vi "Feature Step Call.vi"(11 "Feature List (In)":T2(array[cluster])=[{"Item Name"="test1", "Item Status"=TRUE, "Steps"=[{"Channel Type"="C", "Channels"="6:", "Wait/Poll (ms)"=100, "Parameter"=2, "STM-Speed"=0, "STM-Degree"=0, "Direction"=0}, {"Channel Type"="N", "Channels"="", "Wait/Poll (ms)"=100, "Parameter"=0, "STM-Speed"=0, "STM-Degree"=0, "Direction"=0}, {"Channel Type"="C", "Channels"="6:", "Wait/Poll (ms)"=100, "Parameter"=1, "STM-Speed"=0, "STM-Degree"=0, "Direction"=0}, {"Channel Type"="C", "Channels"="7:", "Wait/Poll (ms)"=100, "Parameter"=2, "STM-Speed"=0, "STM-Degree"=0, "Direction"=0}, {"Channel Type"="C", "Channels"="8:", "Wait/Poll (ms)"=100, "Parameter"=2, "STM-Speed"=0, "STM-Degree"=0, "Direction"=0}, {"Channel Type"="C", "Channels"="7:", "Wait/Poll (ms)"=100, "Parameter"=1, "STM-Speed"=0, "STM-Degree"=0, "Direction"=0}, {"Channel Type"="N", "Channels"="", "Wait/Poll (ms)"=100, "Parameter"=0, "STM-Speed"=0, "STM-Degree"=0, "Direction"=0}]}, {"Item Name"="test2", "Item Status"=TRUE, "Steps"=[{"Channel Type"="C", "Channels"="11:", "Wait/Poll (ms)"=100, "Parameter"=2, "STM-Speed"=0, "STM-Degree"=0, "Direction"=0}, {"Channel Type"="C", "Channels"="12:", "Wait/Poll (ms)"=100, "Parameter"=1, "STM-Speed"=0, "STM-Degree"=0, "Direction"=0}, {"Channel Type"="C", "Channels"="12:", "Wait/Poll (ms)"=100, "Parameter"=2, "STM-Speed"=0, "STM-Degree"=0, "Direction"=0}, {"Channel Type"="C", "Channels"="12:", "Wait/Poll (ms)"=100, "Parameter"=1, "STM-Speed"=0, "STM-Degree"=0, "Direction"=0}, {"Channel Type"="N", "Channels"="", "Wait/Poll (ms)"=100, "Parameter"=0, "STM-Speed"=0, "STM-Degree"=0, "Direction"=0}]}]) -> (0 "Feature Step":string[][](array[string]), 1 "Feature list out":T2(array[cluster]))   [LabVIEW 2015]
uses:
  Galobal variable_TI.vi
panel:
  out "Channels (Out)":i32[](array[numeric])
  out "Channels":string
  out "Feature list out 2":T1(array[cluster])=[{"Item Name"="Winker", "Item Status"=TRUE, "Steps"=[{"Channel Type"="C", "Channels"="3:", "Wait/Poll (ms)"=0, "Parameter"=2, "STM-Speed"=0, "STM-Degree"=0, "Direction"=0}, {"Channel Type"="N", "Channels"="", "Wait/Poll (ms)"=500, "Parameter"=0, "STM-Speed"=0, "STM-Degree"=0, "Direction"=0}, {"Channel Type"="AI", "Channels"="5:", "Wait/Poll (ms)"=1000, "Parameter"=2, "STM-Speed"=0, "STM-Degree"=0, "Direction"=0}, {"Channel Type"="AI", "Channels"="0:", "Wait/Poll (ms)"=1000, "Parameter"=2, "STM-Speed"=0, "STM-Degree"=0, "Direction"=0}, {"Channel Type"="N", "Channels"="", "Wait/Poll (ms)"=500, "Parameter"=0, "STM-Speed"=0, "STM-Degree"=0, "Direction"=0}, {"Channel Type"="C", "Channels"="3:", "Wait/Poll (ms)"=0, "Parameter"=1, "STM-Speed"=0, "STM-Degree"=0, "Direction"=0}, {"Channel Type"="N", "Channels"="", "Wait/Poll (ms)"=500, "Parameter"=0, "STM-Speed"=0, "STM-Degree"=0, "Direction"=0}, {"Channel Type"="N", "Channels"="", "Wait/Poll (ms)"=500, "Parameter"=0, "STM-Speed"=0, "STM-Degree"=0, "Direction"=0}, {"Channel Type"="C", "Channels"="5:", "Wait/Poll (ms)"=0, "Parameter"=2, "STM-Speed"=0, "STM-Degree"=0, "Direction"=0}, {"Channel Type"="C", "Channels"="5:", "Wait/Poll (ms)"=0, "Parameter"=1, "STM-Speed"=0, "STM-Degree"=0, "Direction"=0}, {"Channel Type"="N", "Channels"="", "Wait/Poll (ms)"=500, "Parameter"=0, "STM-Speed"=0, "STM-Degree"=0, "Direction"=0}, {"Channel Type"="N", "Channels"="", "Wait/Poll (ms)"=500, "Parameter"=0, "STM-Speed"=0, "STM-Degree"=0, "Direction"=0}, {"Channel Type"="N", "Channels"="", "Wait/Poll (ms)"=500, "Parameter"=0, "STM-Speed"=0, "STM-Degree"=0, "Direction"=0}, {"Channel Type"="C", "Channels"="4:", "Wait/Poll (ms)"=0, "Parameter"=2, "STM-Speed"=0, "STM-Degree"=0, "Direction"=0}, {"Channel Type"="N", "Channels"="", "Wait/Poll (ms)"=500, "Parameter"=0, "STM-Speed"=0, "STM-Degree"=0, "Direction"=0}, {"Channel Type"="AI", "Channels"="4:", "Wait/Poll (ms)"=1000, "Parameter"=2, "STM-Speed"=0, "STM-Degree"=0, "Direction"=0}, {"Channel Type"="AI", "Channels"="0:", "Wait/Poll (ms)"=1000, "Parameter"=2, "STM-Speed"=0, "STM-Degree"=0, "Direction"=0}, {"Channel Type"="N", "Channels"="", "Wait/Poll (ms)"=500, "Parameter"=0, "STM-Speed"=0, "STM-Degree"=0, "Direction"=0}, {"Channel Type"="C", "Channels"="4:", "Wait/Poll (ms)"=0, "Parameter"=1, "STM-Speed"=0, "STM-Degree"=0, "Direction"=0}, {"Channel Type"="N", "Channels"="", "Wait/Poll (ms)"=500, "Parameter"=0, "STM-Speed"=0, "STM-Degree"=0, "Direction"=0}, {"Channel Type"="N", "Channels"="", "Wait/Poll (ms)"=500, "Parameter"=0, "STM-Speed"=0, "STM-Degree"=0, "Direction"=0}, {"Channel Type"="C", "Channels"="5:", "Wait/Poll (ms)"=0, "Parameter"=2, "STM-Speed"=0, "STM-Degree"=0, "Direction"=0}, {"Channel Type"="N", "Channels"="", "Wait/Poll (ms)"=500, "Parameter"=0, "STM-Speed"=0, "STM-Degree"=0, "Direction"=0}, {"Channel Type"="N", "Channels"="", "Wait/Poll (ms)"=500, "Parameter"=0, "STM-Speed"=0, "STM-Degree"=0, "Direction"=0}, {"Channel Type"="C", "Channels"="5:", "Wait/Poll (ms)"=0, "Parameter"=1, "STM-Speed"=0, "STM-Degree"=0, "Direction"=0}, {"Channel Type"="N", "Channels"="", "Wait/Poll (ms)"=500, "Parameter"=0, "STM-Speed"=0, "STM-Degree"=0, "Direction"=0}, {"Channel Type"="N", "Channels"="", "Wait/Poll (ms)"=500, "Parameter"=0, "STM-Speed"=0, "STM-Degree"=0, "Direction"=0}]}, {"Item Name"="Horn", "Item Status"=TRUE, "Steps"=[{"Channel Type"="C", "Channels"="8:", "Wait/Poll (ms)"=0, "Parameter"=2, "STM-Speed"=0, "STM-Degree"=0, "Direction"=0}, {"Channel Type"="N", "Channels"="", "Wait/Poll (ms)"=500, "Parameter"=0, "STM-Speed"=0, "STM-Degree"=0, "Direction"=0}, {"Channel Type"="AI", "Channels"="9:", "Wait/Poll (ms)"=1000, "Parameter"=2, "STM-Speed"=0, "STM-Degree"=0, "Direction"=0}, {"Channel Type"="AI", "Channels"="3:", "Wait/Poll (ms)"=1000, "Parameter"=2, "STM-Speed"=0, "STM-Degree"=0, "Direction"=0}, {"Channel Type"="N", "Channels"="", "Wait/Poll (ms)"=500, "Parameter"=0, "STM-Speed"=0, "STM-Degree"=0, "Direction"=0}, {"Channel Type"="C", "Channels"="8:", "Wait/Poll (ms)"=0, "Parameter"=1, "STM-Speed"=0, "STM-Degree"=0, "Direction"=0}, {"Channel Type"="N", "Channels"="", "Wait/Poll (ms)"=500, "Parameter"=0, "STM-Speed"=0, "STM-Degree"=0, "Direction"=0}, {"Channel Type"="N", "Channels"="", "Wait/Poll (ms)"=500, "Parameter"=0, "STM-Speed"=0, "STM-Degree"=0, "Direction"=0}]}, {"Item Name"="Passing", "Item Status"=TRUE, "Steps"=[{"Channel Type"="C", "Channels"="8:", "Wait/Poll (ms)"=0, "Parameter"=2, "STM-Speed"=0, "STM-Degree"=0, "Direction"=0}, {"Channel Type"="N", "Channels"="", "Wait/Poll (ms)"=500, "Parameter"=0, "STM-Speed"=0, "STM-Degree"=0, "Direction"=0}, {"Channel Type"="C", "Channels"="8:", "Wait/Poll (ms)"=0, "Parameter"=1, "STM-Speed"=0, "STM-Degree"=0, "Direction"=0}, {"Channel Type"="N", "Channels"="", "Wait/Poll (ms)"=500, "Parameter"=0, "STM-Speed"=0, "STM-Degree"=0, "Direction"=0}]}, {"Item Name"="-1", "Item Status"=FALSE, "Steps"=[]}, {"Item Name"="-1", "Item Status"=FALSE, "Steps"=[]}, {"Item Name"="-1", "Item Status"=FALSE, "Steps"=[]}, {"Item Name"="-1", "Item Status"=FALSE, "Steps"=[]}, {"Item Name"="Screw ", "Item Status"=TRUE, "Steps"=[{"Channel Type"="C", "Channels"="1:", "Wait/Poll (ms)"=1000, "Parameter"=1, "STM-Speed"=0, "STM-Degree"=0, "Direction"=0}, {"Channel Type"="F", "Channels"="12:", "Wait/Poll (ms)"=1000, "Parameter"=1, "STM-Speed"=0, "STM-Degree"=0, "Direction"=0}, {"Channel Type"="C", "Channels"="0:", "Wait/Poll (ms)"=1000, "Parameter"=2, "STM-Speed"=0, "STM-Degree"=0, "Direction"=0}, {"Channel Type"="N", "Channels"="", "Wait/Poll (ms)"=200, "Parameter"=0, "STM-Speed"=0, "STM-Degree"=0, "Direction"=0}, {"Channel Type"="F", "Channels"="12:", "Wait/Poll (ms)"=1000, "Parameter"=2, "STM-Speed"=0, "STM-Degree"=0, "Direction"=0}, {"Channel Type"="N", "Channels"="", "Wait/Poll (ms)"=200, "Parameter"=0, "STM-Speed"=0, "STM-Degree"=0, "Direction"=0}, {"Channel Type"="C", "Channels"="0:", "Wait/Poll (ms)"=0, "Parameter"=1, "STM-Speed"=0, "STM-Degree"=0, "Direction"=0}, {"Channel Type"="N", "Channels"="", "Wait/Poll (ms)"=100, "Parameter"=0, "STM-Speed"=0, "STM-Degree"=0, "Direction"=0}]}, {"Item Name"="Stamping", "Item Status"=TRUE, "Steps"=[{"Channel Type"="C", "Channels"="5:", "Wait/Poll (ms)"=1000, "Parameter"=2, "STM-Speed"=0, "STM-Degree"=0, "Direction"=0}, {"Channel Type"="N", "Channels"="", "Wait/Poll (ms)"=200, "Parameter"=0, "STM-Speed"=0, "STM-Degree"=0, "Direction"=0}, {"Channel Type"="F", "Channels"="13:", "Wait/Poll (ms)"=1000, "Parameter"=2, "STM-Speed"=0, "STM-Degree"=0, "Direction"=0}, {"Channel Type"="C", "Channels"="5:", "Wait/Poll (ms)"=1000, "Parameter"=1, "STM-Speed"=0, "STM-Degree"=0, "Direction"=0}, {"Channel Type"="C", "Channels"="6:", "Wait/Poll (ms)"=1000, "Parameter"=2, "STM-Speed"=0, "STM-Degree"=0, "Direction"=0}, {"Channel Type"="N", "Channels"="", "Wait/Poll (ms)"=200, "Parameter"=0, "STM-Speed"=0, "STM-Degree"=0, "Direction"=0}, {"Channel Type"="F", "Channels"="14:", "Wait/Poll (ms)"=1000, "Parameter"=2, "STM-Speed"=0, "STM-Degree"=0, "Direction"=0}, {"Channel Type"="C", "Channels"="6:", "Wait/Poll (ms)"=1000, "Parameter"=1, "STM-Speed"=0, "STM-Degree"=0, "Direction"=0}, {"Channel Type"="N", "Channels"="", "Wait/Poll (ms)"=200, "Parameter"=0, "STM-Speed"=0, "STM-Degree"=0, "Direction"=0}]}, {"Item Name"="Screw off", "Item Status"=TRUE, "Steps"=[{"Channel Type"="C", "Channels"="0:", "Wait/Poll (ms)"=0, "Parameter"=1, "STM-Speed"=0, "STM-Degree"=0, "Direction"=0}, {"Channel Type"="C", "Channels"="1:", "Wait/Poll (ms)"=0, "Parameter"=2, "STM-Speed"=0, "STM-Degree"=0, "Direction"=0}, {"Channel Type"="N", "Channels"="", "Wait/Poll (ms)"=100, "Parameter"=0, "STM-Speed"=0, "STM-Degree"=0, "Direction"=0}, {"Channel Type"="N", "Channels"="", "Wait/Poll (ms)"=500, "Parameter"=0, "STM-Speed"=0, "STM-Degree"=0, "Direction"=0}, {"Channel Type"="N", "Channels"="", "Wait/Poll (ms)"=100, "Parameter"=0, "STM-Speed"=0, "STM-Degree"=0, "Direction"=0}, {"Channel Type"="F", "Channels"="12:", "Wait/Poll (ms)"=1000, "Parameter"=1, "STM-Speed"=0, "STM-Degree"=0, "Direction"=0}, {"Channel Type"="C", "Channels"="0:", "Wait/Poll (ms)"=1000, "Parameter"=1, "STM-Speed"=0, "STM-Degree"=0, "Direction"=0}, {"Channel Type"="N", "Channels"="", "Wait/Poll (ms)"=100, "Parameter"=0, "STM-Speed"=0, "STM-Degree"=0, "Direction"=0}]}, {"Item Name"="Reset", "Item Status"=TRUE, "Steps"=[{"Channel Type"="C", "Channels"="2:", "Wait/Poll (ms)"=0, "Parameter"=1, "STM-Speed"=0, "STM-Degree"=0, "Direction"=0}, {"Channel Type"="N", "Channels"="", "Wait/Poll (ms)"=50, "Parameter"=0, "STM-Speed"=0, "STM-Degree"=0, "Direction"=0}, {"Channel Type"="C", "Channels"="3:", "Wait/Poll (ms)"=0, "Parameter"=1, "STM-Speed"=0, "STM-Degree"=0, "Direction"=0}, {"Channel Type"="N", "Channels"="", "Wait/Poll (ms)"=50, "Parameter"=0, "STM-Speed"=0, "STM-Degree"=0, "Direction"=0}, {"Channel Type"="C", "Channels"="4:", "Wait/Poll (ms)"=0, "Parameter"=1, "STM-Speed"=0, "STM-Degree"=0, "Direction"=0}, {"Channel Type"="N", "Channels"="", "Wait/Poll (ms)"=50, "Parameter"=0, "STM-Speed"=0, "STM-Degree"=0, "Direction"=0}, {"Channel Type"="C", "Channels"="7:", "Wait/Poll (ms)"=0, "Parameter"=1, "STM-Speed"=0, "STM-Degree"=0, "Direction"=0}, {"Channel Type"="N", "Channels"="", "Wait/Poll (ms)"=50, "Parameter"=0, "STM-Speed"=0, "STM-Degree"=0, "Direction"=0}, {"Channel Type"="C", "Channels"="8:", "Wait/Poll (ms)"=0, "Parameter"=1, "STM-Speed"=0, "STM-Degree"=0, "Direction"=0}, {"Channel Type"="N", "Channels"="", "Wait/Poll (ms)"=50, "Parameter"=0, "STM-Speed"=0, "STM-Degree"=0, "Direction"=0}, {"Channel Type"="C", "Channels"="9:", "Wait/Poll (ms)"=0, "Parameter"=1, "STM-Speed"=0, "STM-Degree"=0, "Direction"=0}, {"Channel Type"="N", "Channels"="", "Wait/Poll (ms)"=50, "Parameter"=0, "STM-Speed"=0, "STM-Degree"=0, "Direction"=0}, {"Channel Type"="C", "Channels"="12:", "Wait/Poll (ms)"=0, "Parameter"=1, "STM-Speed"=0, "STM-Degree"=0, "Direction"=0}, {"Channel Type"="N", "Channels"="", "Wait/Poll (ms)"=50, "Parameter"=0, "STM-Speed"=0, "STM-Degree"=0, "Direction"=0}, {"Channel Type"="C", "Channels"="0:", "Wait/Poll (ms)"=0, "Parameter"=1, "STM-Speed"=0, "STM-Degree"=0, "Direction"=0}, {"Channel Type"="N", "Channels"="", "Wait/Poll (ms)"=50, "Parameter"=0, "STM-Speed"=0, "STM-Degree"=0, "Direction"=0}, {"Channel Type"="C", "Channels"="1:", "Wait/Poll (ms)"=0, "Parameter"=2, "STM-Speed"=0, "STM-Degree"=0, "Direction"=0}, {"Channel Type"="N", "Channels"="", "Wait/Poll (ms)"=50, "Parameter"=0, "STM-Speed"=0, "STM-Degree"=0, "Direction"=0}, {"Channel Type"="N", "Channels"="", "Wait/Poll (ms)"=50, "Parameter"=0, "STM-Speed"=0, "STM-Degree"=0, "Direction"=0}, {"Channel Type"="C", "Channels"="1:", "Wait/Poll (ms)"=0, "Parameter"=1, "STM-Speed"=0, "STM-Degree"=0, "Direction"=0}, {"Channel Type"="N", "Channels"="", "Wait/Poll (ms)"=100, "Parameter"=0, "STM-Speed"=0, "STM-Degree"=0, "Direction"=0}]}]
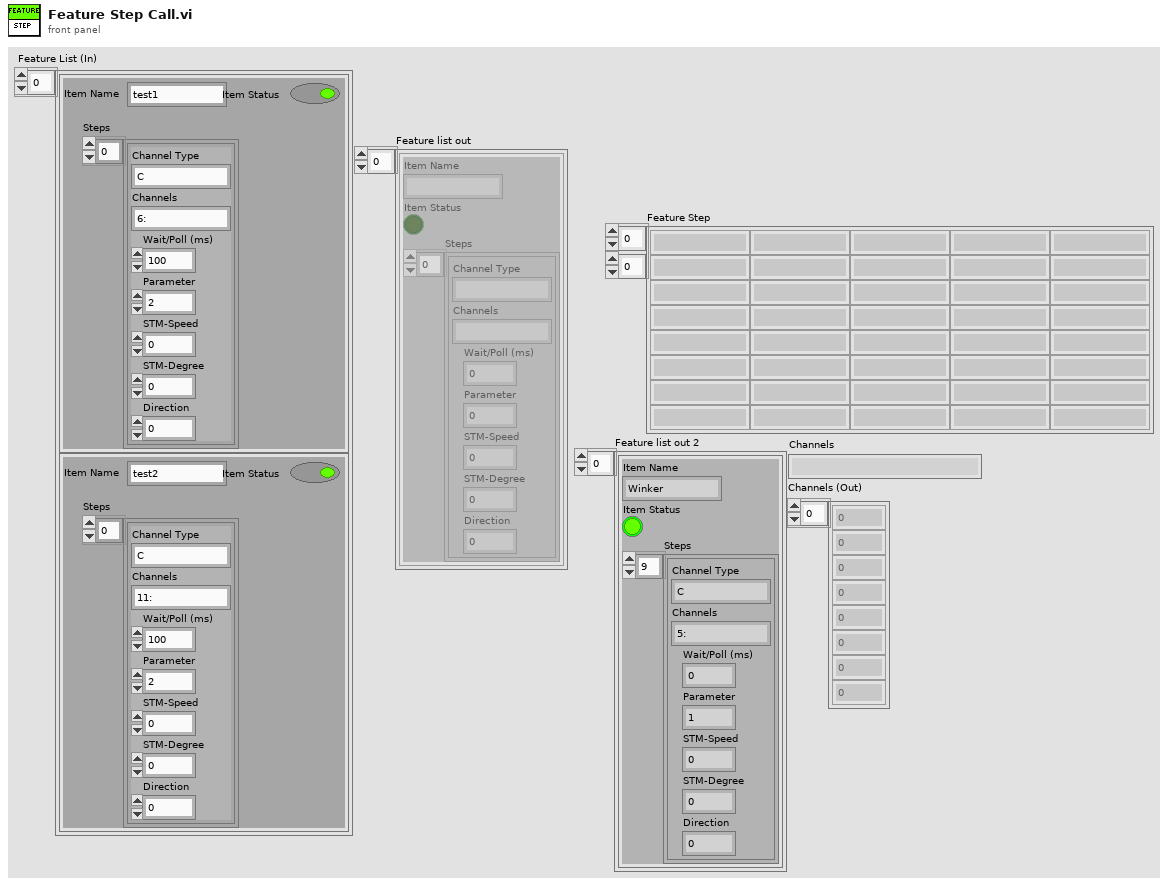
[diagram p1: front panel]
types:
  T1 = cluster{"Item Name":string, "Item Status":bool, "Steps":cluster{"Channel Type":string, "Channels":string, "Wait/Poll (ms)":u32, "Parameter":u8, "STM-Speed":u8, "STM-Degree":u32, "Direction":u8}[]}[]
  T2 = cluster{"Item Name":string, "Item Status":bool, "Steps":cluster{"Channel Type":string, "Channels":string, "Wait/Poll (ms)":u32, "Parameter":u8, "STM-Speed":i32, "STM-Degree":u32, "Direction":u8}[]}[]
  T3 = cluster{"Item Name":string, "Item Status":bool, "Steps":cluster{"Channel Type":string, "Channels":string, "Wait/Poll (ms)":u32, "Parameter":u8, "STM-Speed":u8, "STM-Degree":u32, "Direction":u8}[]}
  T4 = cluster{"Channel Type":string, "Channels":string, "Wait/Poll (ms)":u32, "Parameter":u8, "STM-Speed":u8, "STM-Degree":u32, "Direction":u8}[]
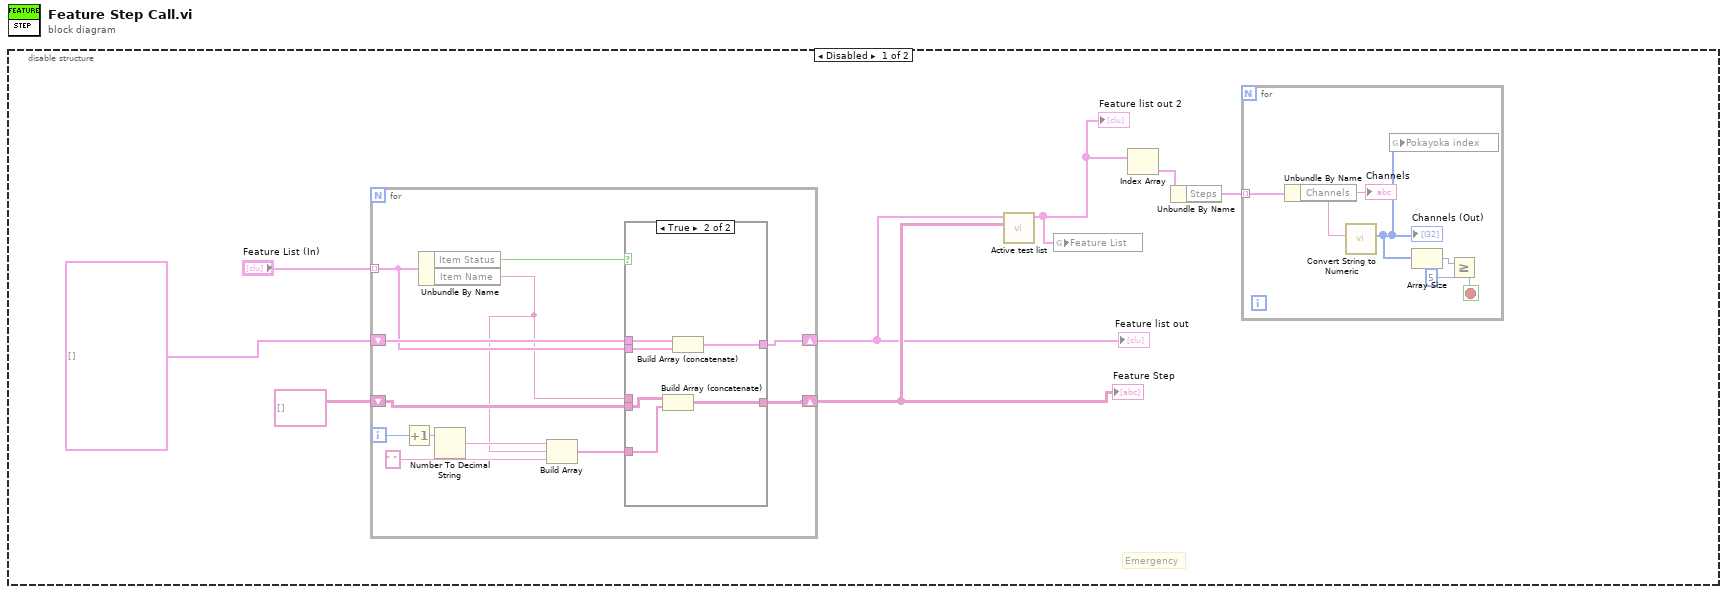
[diagram p0: block diagram]
diagram:
  n1 = disable-structure shown="Disabled" {
    frame Disabled {
      # "Emergency"
      n2 = for {
        tunnel: "Feature List (In)" -> [w23] mode=indexing
        shift-right: [w25] -> w1
        shift-left: T2 [] ("Array") -> [w24]
        shift-right: [w22] -> w2
        shift-left: string[][] [] -> [w21]
        i -> [w19]
        n3 = Increment(x=w19) -> (x+1=w20:i32)
        n4 = Unbundle By Name(w23) -> ("Item Status"=w26:bool, "Item Name"=w17:string)
        n5 = Number To Decimal String(number=w20) -> (decimal integer string=w18:string)  [unwired: 1 in]
        n6 = Build Array(w18, w17, " ") -> (w15:string[])
        n7 = case shown="True" w26 {
          tunnel: w23 -> [_ w31]
          tunnel: [w28 w34] -> w25
          tunnel: w24 -> [w28 w32]
          tunnel: w17 -> [_ _]
          tunnel: [w27 w33] -> w22
          tunnel: w21 -> [w27 w30]
          tunnel: w15 -> [_ w29]
          frame False {
          }
          frame True {
            n8 = Build Array (concatenate)(w30, w29) -> (w33:string[][])
            n9 = Build Array (concatenate)(w32, w31) -> (w34:T2)
          }
        }
      }
      "Feature Step" <- w2
      "Feature list out" <- w1
      n10 = call "Active test list.vi"("Feature Step"=w2, "Feature list in"=w1) -> ("Feature list out"=w5:T1)  [unwired: 6 in, 3 out]
      "Feature list out 2" <- w5
      n11 = global write "Galobal variable_TI.vi" "Feature List"(w5) -> ()
      n12 = Index Array(array=w5) -> (element=w4:T3)  [unwired: 1 in]
      n13 = Unbundle By Name(w4) -> ("Steps"=w3:T4)
      n14 = for {
        tunnel: w3 -> [w14] mode=indexing
        stop <- w10 stop-if-true
        n15 = Unbundle By Name(w14) -> ("Channels"=w13:string)
        "Channels" <- w13
        n16 = call "Convert String to Numeric.vi"("Channels (A:B:C:D...) (In)"=w13) -> ("Channels (Out)"=w9:i32[])  [unwired: 9 in, 1 out]
        "Channels (Out)" <- w9
        n17 = global write "Galobal variable_TI.vi" "Pokayoka index"(w9) -> ()
        n18 = Array Size(array=w9) -> (size(s)=w12:i32)
        n19 = Greater Or Equal?(x=w12, y=5) -> (x >= y?=w10:bool)
      }
    }
    frame Enabled {
    }
  }
